vi "1A research - readWindInfo.vi"() -> ()   [LabVIEW 2011]
uses:
  2-Think/2 Typedefs/apparent wind speed.ctl
  2-Think/2 Typedefs/absolute wind direction.ctl
  <vilib>/Utility/file.llb/Write To Spreadsheet File (DBL).vi
  <vilib>/Analysis/3filter.llb/FIR Filter (DBL).vi
  2-Think/2 Globals/2 Global.vi
  <vilib>/Analysis/NI_AALBase.lvlib
  <vilib>/ptbypt/NI_PtbyPt.lvlib
  <vilib>/Utility/file.llb/Read From Spreadsheet File (DBL).vi
panel:
  out "Filtered Wind Speed":dbl
  out "Difference":dbl
  out "element":dbl
  out "Direction, modded":dbl[][](graph)
  out "Waveform Graph 3":dbl[](graph)
  out "subarray":dbl[](array[numeric])
  in  "Frist filter coeff":i32
  out "Direction, unmodded":dbl[][](graph)
  out "Waveform Chart":dbl(graph)
  out "Waveform Graph":dbl[][](graph)
  in  "VISA resource name (in)":refnum<visa-resource-name>="COM1"
  out "Apparent Wind\nDirection":T1
  out "Apparent Wind\nSpeed":T2
  in  "stop":bool
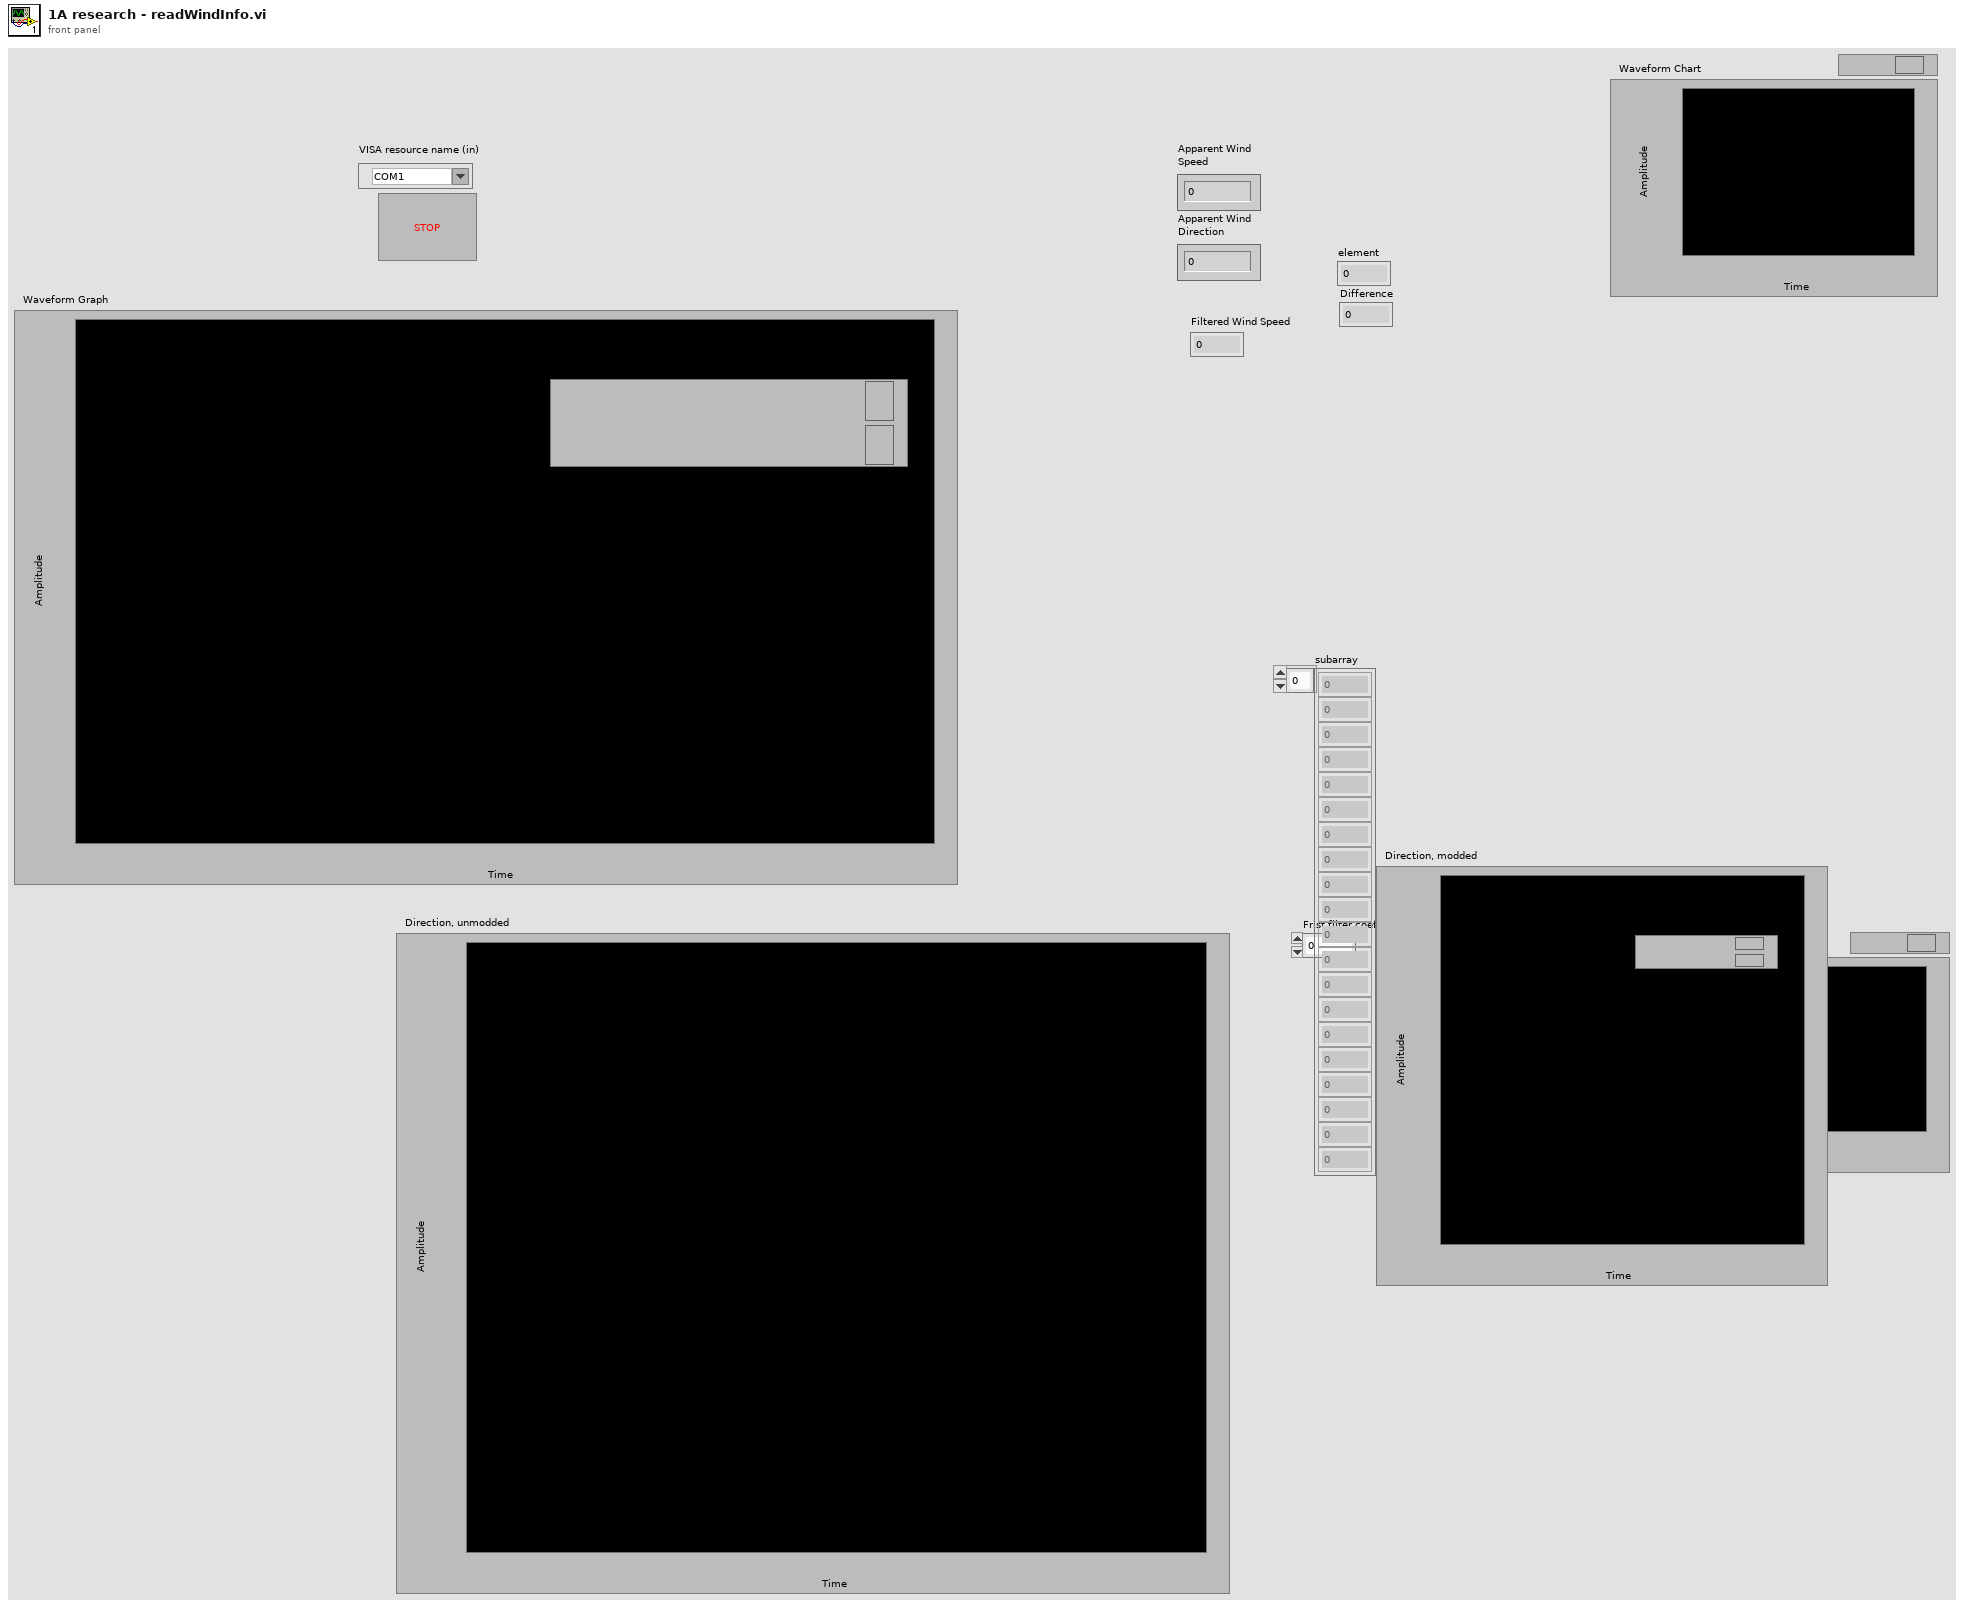
[diagram p1: front panel]
types:
  T1 = typedef "absolute wind direction.ctl" = dbl
  T2 = typedef "apparent wind speed.ctl" = dbl
  T3 = typedef "apparent wind direction.ctl" = dbl
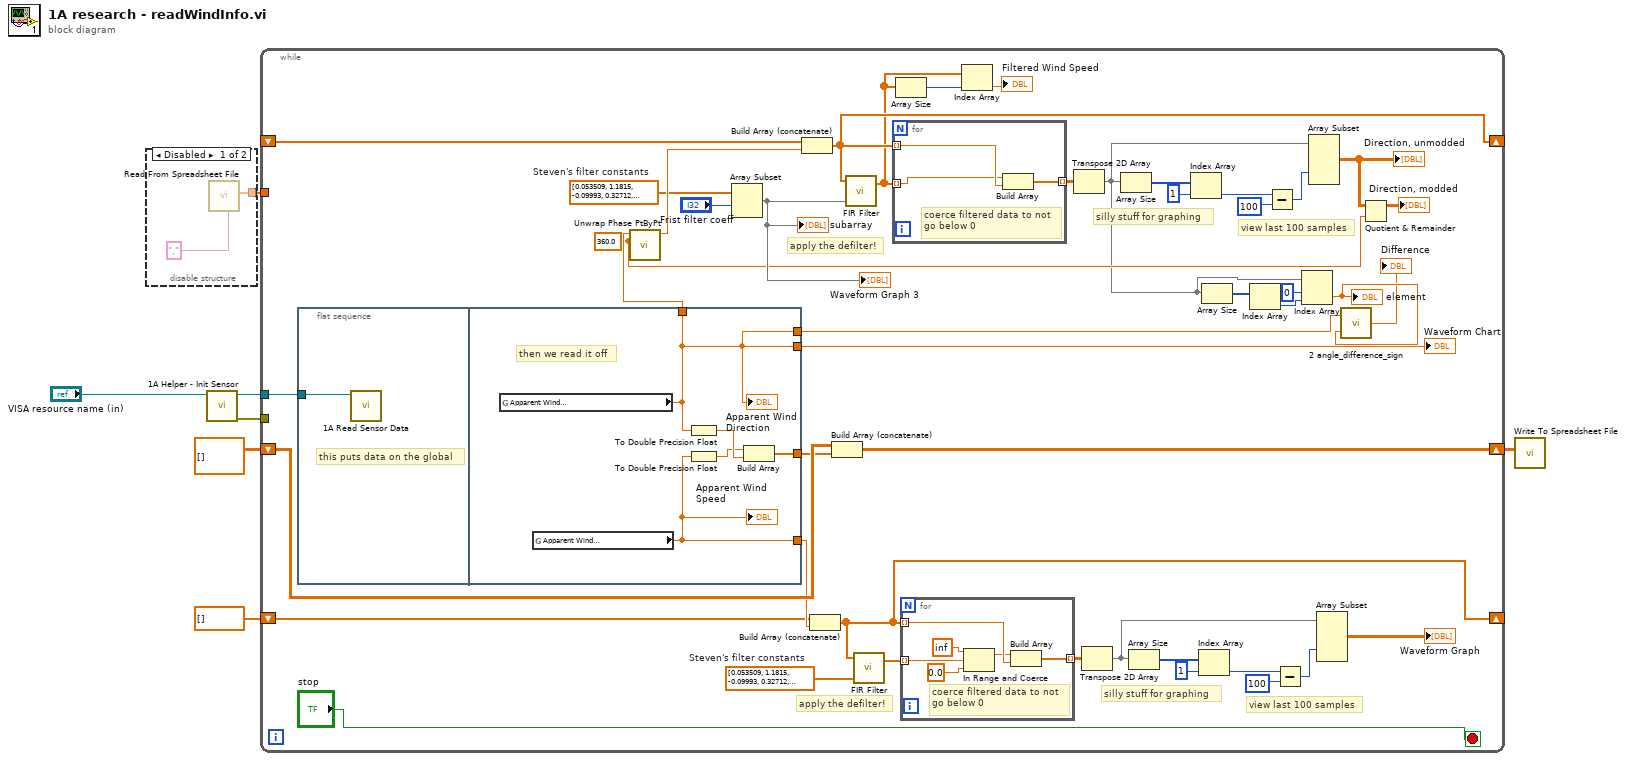
[diagram p0: block diagram]
diagram:
  n1 = disable-structure shown="Disabled" {
    disable-tunnel: [w9 _] -> w1
    frame Disabled {
      n2 = call-poly <vilib>:"Read From Spreadsheet File.vi"("delimiter (\\t)"="," ("delimiter (\\t)")) -> ("first row"=w9:dbl[])  [unwired: 6 in, 4 out]
    }
    frame Enabled {
    }
  }
  n3 = call "1A Helper - Init Sensor.vi"("VISA Refnum in"="VISA resource name (in)") -> ("error out"=w4:errorcluster, "VISA Refnum out"=w5:refnum<visa-resource-name>)  [unwired: 8 in, 1 out]
  n4 = while {
    shift-right: [w50] -> w3
    shift-left: dbl[][] [] -> [w53]
    tunnel: w5 -> [w52]
    tunnel: w4 -> [_]
    shift-right: [w46] -> _
    shift-left: T2[] [] -> [w48]
    shift-right: [w29] -> _
    shift-left: _ -> [w30]
    tunnel: w1 -> [_]
    stop <- "stop" stop-if-true
    w13 = dbl[] [0.053509, 1.1815, -0.09993, 0.32712, 0.10938, 0.11358, 0.13924, -0.16172, 0.45069, -0.055441, 0.019471, 0.082764, 0.12364, -0.39235, -0.19677, 0.3546, 0.16406, -0.070202, -0.10287, -0.028649, 0.018791, -0.038948, 0.097859, -0.0038871, -0.027341, 0.025466, 0.10393, -0.25443, 0.039379, -0.052109, -0.089114, 0.018497, -0.76719, 0.10647, -0.024919, -0.062391, 0.024126, 0.47711, -1.0783, 0.17365, 0.32185, 0.30825, 0.069773, 0.0316, -0.81283, -0.038254, 0.1407, 0.043989, 0.064417, 0.051313, 0.19402, -0.16605]  # Steven's filter constants
    w22 = 360.0 ("wrap base")
    w21 = dbl[] [0.053509, 1.1815, -0.09993, 0.32712, 0.10938, 0.11358, 0.13924, -0.16172, 0.45069, -0.055441, 0.019471, 0.082764, 0.12364, -0.39235, -0.19677, 0.3546, 0.16406, -0.070202, -0.10287, -0.028649, 0.018791, -0.038948, 0.097859, -0.0038871, -0.027341, 0.025466, 0.10393, -0.25443, 0.039379, -0.052109, -0.089114, 0.018497, -0.76719, 0.10647, -0.024919, -0.062391, 0.024126, 0.47711, -1.0783, 0.17365, 0.32185, 0.30825, 0.069773, 0.0316, -0.81283, -0.038254, 0.1407, 0.043989, 0.064417, 0.051313, 0.19402, -0.16605]  # Steven's filter constants
    # "view last 100 samples"
    # "silly stuff for graphing"
    # "apply the defilter!"
    # "view last 100 samples"
    # "silly stuff for graphing"
    # "apply the defilter!"
    n5 = flat-sequence {
      tunnel: w52 -> [w64]
      tunnel: [w68] -> w51
      tunnel: [w66] -> w49
      tunnel: [w65] -> w37
      tunnel: [w65] -> w28
      tunnel: [w65] -> w17
      frame #0 {
        # "this puts data on the global"
        n6 = call "1A Read Sensor Data.vi"("VISA resource name (in)"=w64) -> ()  [unwired: 9 in, 2 out]
      }
      frame #1 {
        # "then we read it off"
        n7 = global read "2 Global.vi" "Apparent Wind\nDirection (º)"() -> (w65:T3)
        "Apparent Wind\nDirection" <- w65
        n8 = global read "2 Global.vi" "Apparent Wind\nSpeed"() -> (w66:T2)
        "Apparent Wind\nSpeed" <- w66
        n9 = To Double Precision Float(number=w65) -> (double precision float=w69:T3)
        n10 = To Double Precision Float(number=w66) -> (double precision float=w67:T2)
        n11 = Build Array(w67, w69) -> (w68:T3[])
      }
    }
    n12 = call <vilib>:"Unwrap Phase PtByPt.vi"("wrap base"=w22, "phase"=w28) -> ("unwrapped phase"=w27:dbl)  [unwired: 9 in]
    n13 = Array Subset(array=w13, index="Frist filter coeff") -> (w25:dbl[])  [unwired: 1 in]
    "subarray" <- w25
    "Waveform Graph 3" <- w25
    n14 = Build Array (concatenate)(w30, w27) -> (w29:dbl[])
    n15 = Build Array (concatenate)(w48, w49) -> (w46:T2[])
    n16 = Build Array (concatenate)(w53, w51) -> (w50:T3[][])
    n17 = call-poly <vilib>:"FIR Filter.vi"("FIR Coefficients"=w25, "X"=w29) -> ("Filtered X"=w12:dbl[])  [unwired: 2 in, 1 out]
    n18 = call-poly <vilib>:"FIR Filter.vi"("FIR Coefficients"=w21, "X"=w46) -> ("Filtered X"=w47:dbl[])  [unwired: 2 in, 1 out]
    n19 = for {
      tunnel: w29 -> [w56] mode=indexing
      tunnel: w12 -> [w55] mode=indexing
      tunnel: [w57] -> w31 mode=indexing
      # "coerce filtered data to not\ngo below 0"
      n20 = Build Array(w55, w56) -> (w57:dbl[])
    }
    n21 = Array Size(array=w12) -> (size(s)=w11:i32)
    n22 = for {
      tunnel: w46 -> [w59] mode=indexing
      tunnel: w47 -> [w62] mode=indexing
      tunnel: [w63] -> w45 mode=indexing
      # "coerce filtered data to not\ngo below 0"
      n23 = In Range and Coerce(upper limit=inf, x=w62, lower limit=0.0) -> (coerced(x)=w58:dbl)  [unwired: 1 out]
      n24 = Build Array(w58, w59) -> (w63:T2[])
    }
    n25 = Index Array(array=w12, index=w11) -> (element=→"Filtered Wind Speed":dbl)
    n26 = Transpose 2D Array(2D array=w31) -> (transposed array=w20:dbl[][])
    n27 = Transpose 2D Array(2D array=w45) -> (transposed array=w44:T2[][])
    n28 = Array Size(array=w20) -> (size(s)=w33:i32[])
    n29 = Array Size(array=w44) -> (size(s)=w42:i32[])
    n30 = Index Array(array=w33, index=1) -> (element=w34:i32)
    n31 = Index Array(array=w42, index=1) -> (element=w41:i32)
    n32 = Array Size(array=w20) -> (size(s)=w19:i32[])
    n33 = Index Array(array=w19) -> (element=w18:i32)  [unwired: 1 in]
    n34 = Subtract(x=w34, y=100) -> (x-y=w36:i32)
    n35 = Subtract(x=w41, y=100) -> (x-y=w39:i32)
    n36 = Index Array(array=w20, index (row)=0 ("disabled index (row)"), index (col)=w18) -> (element=w15:dbl)
    "element" <- w15
    n37 = Array Subset(array=w20, index (col)=w36) -> (w23:dbl[][])  [unwired: 3 in]
    "Direction, unmodded" <- w23
    n38 = Array Subset(array=w44, index (col)=w39) -> (→"Waveform Graph":T2[][])  [unwired: 3 in]
    n39 = call "2 angle_difference_sign.vi"("Angle 2"=w15, "Angle 1"=w17) -> ("Difference"=→"Difference":dbl)
    n40 = Quotient & Remainder(x=w23, y=w22) -> (x-y*floor(x/y)=→"Direction, modded":dbl[][])  [unwired: 1 out]
    "Waveform Chart" <- w37
  }
  n41 = call-poly <vilib>:"Write To Spreadsheet File.vi"("2D data"=w3) -> ()  [unwired: 7 in, 1 out]
